vi "GA Get Gear Ratio.vi"(0 "nAxisNum":i16, 1 "pStopSmoothTime":i32, 5 "pMasterEven":i32, 7 "pSlaveEven":i32, 9 "pMasterSlope":i32, 11 "error in (no error)":errorcluster caption="错误输入（无错误）") -> (3 "pStopSmoothTime out":i32, 4 "function return":i32, 6 "pMasterEven out":i32, 8 "pSlaveEven out":i32, 10 "pMasterSlope out":i32, 15 "error out":errorcluster caption="错误输出")   [LabVIEW 2015, in "GAS.lvlib"]
doc: "extern \"C\" __declspec(dllimport) int GA_GetGearRatio(short nAxisNum,long *pMasterEven,long *pSlaveEven,long *pMasterSlope=NULL,long *pStopSmoothTime=NULL);"
uses:
  <userlib>/BP_GAS/GAS.lvlib
  <userlib>/BP_GAS/GAS.dll
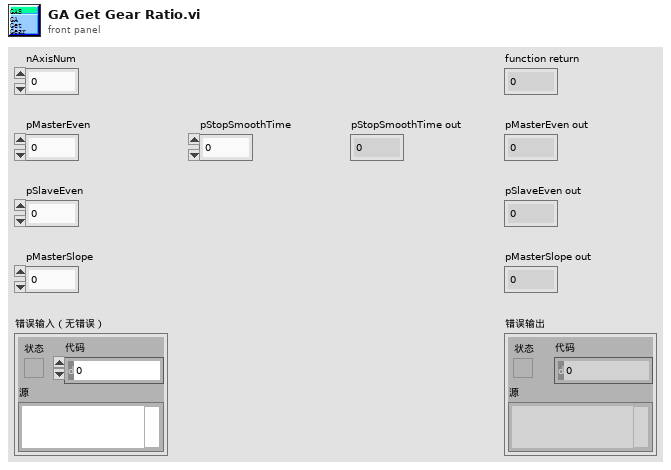
[diagram p1: front panel]
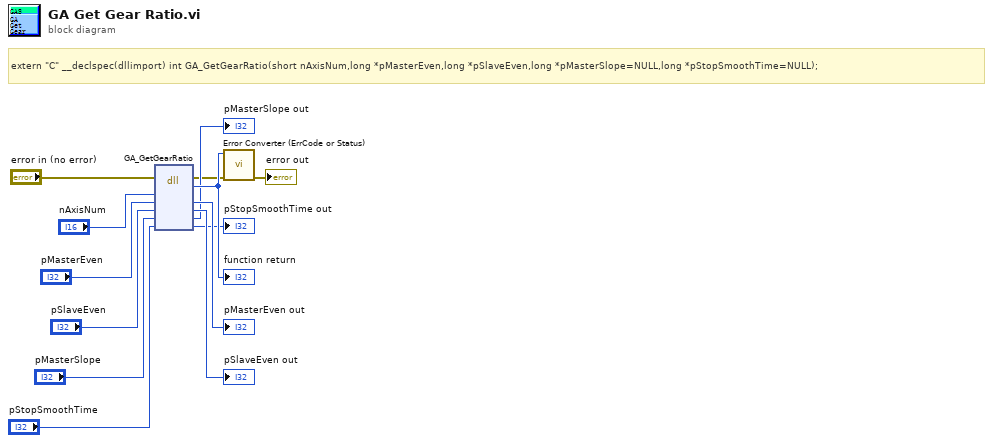
[diagram p0: block diagram]
diagram:
  # "extern \"C\" __declspec(dllimport) int GA_GetGearRatio(short nAxisNum,long *pMasterEven,long *pSlaveEven,long *pMasterSlope=NULL,long *pStopSmoothTime=NULL);"
  n1 = dll-call lib="E:/Program Files (x86)/National Instruments/LabVIEW 2015/user.lib/BP_GAS/GAS.*" fn="GA_GetGearRatio"(error in="error in (no error)", "nAxisNum"="nAxisNum", "pMasterEven"="pMasterEven", "pSlaveEven"="pSlaveEven", "pMasterSlope"="pMasterSlope", "pStopSmoothTime"="pStopSmoothTime") -> (error out=w2:errorcluster, w13:i32, "pMasterEven"=→"pMasterEven out":i32, "pSlaveEven"=→"pSlaveEven out":i32, "pMasterSlope"=→"pMasterSlope out":i32, "pStopSmoothTime"=→"pStopSmoothTime out":i32)  [unwired: 3 in, 1 out]
  "function return" <- w13
  n2 = call "Error Converter (ErrCode or Status).vi"("error in (no error)"=w2, "error code"=w13) -> ("error out"=→"error out":errorcluster)  [unwired: 9 in]
